vi "Control - Diesel - Cranking Host.vi"() -> ()   [LabVIEW 2015, in "ECS-Host.lvlib"]
uses:
  ECS-Host.lvlib
  <vilib>/addons/Software Calibration Management/XControls/TBL2D.xctl
panel:
  out "EngineStatus":u8
  out "_EngineStatus":enum32{"STALLED", "CRANKING", "RUNNING"}(ring)
  out "CrankModeActive":bool
  in  "ForceCrank_E":bool
  in  "Crank_E":bool
  in  "_LUT Tab":T1(tab)
  in  "InjTiming_ManE":bool
  out "InjTiming_TblOut":sgl caption="[]"
  in  "InjTiming_Man":sgl caption="[]"
  in  "InjTiming_Tbl":cluster{"X":sgl[], "Y":sgl[], "Z":sgl[][]}(xcontrol) caption="[]"
  out "InjQty_Calc":sgl caption="[]"
  in  "Phi_Max":sgl caption="[]"
  in  "InjQty_ManE":bool
  out "InjQty_TblOut":sgl caption="[]"
  in  "InjQty_Man":sgl caption="[]"
  in  "InjQty_Tbl":cluster{"X":sgl[], "Y":sgl[], "Z":sgl[][]}(xcontrol) caption="[]"
  in  "RailP_ManE":bool
  out "RailP_TblOut":sgl caption="[]"
  in  "RailP_Man":sgl caption="[]"
  in  "RailP_Tbl":cluster{"X":sgl[], "Y":sgl[], "Z":sgl[][]}(xcontrol) caption="[]"
  in  "VVTCam1Adv_ManE":bool
  out "VVTCam1Adv_TblOut":sgl caption="[]"
  in  "VVTCam1Adv_Man":sgl caption="[]"
  in  "VVTCam1Adv_Tbl":cluster{"X":sgl[], "Y":sgl[], "Z":sgl[][]}(xcontrol) caption="[]"
  in  "VVTCam2Adv_ManE":bool
  out "VVTCam2Adv_TblOut":sgl caption="[]"
  in  "VVTCam2Adv_Man":sgl caption="[]"
  in  "VVTCam2Adv_Tbl":cluster{"X":sgl[], "Y":sgl[], "Z":sgl[][]}(xcontrol) caption="[]"
  in  "VGTPsn_Crank":sgl caption="[%Open]"
  in  "WgPsn_Crank":sgl caption="[%Open]"
  in  "LowPEGRPsn_Crank":sgl caption="[%Open]"
  in  "HighPEGRPsn_Crank":sgl caption="[%Open]"
  # "(Smoke Limit)"
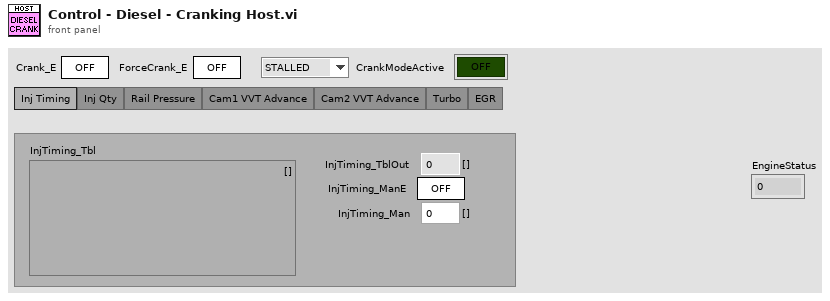
[diagram p1: front panel]
types:
  T1 = enum32{"Inj Timing", "Inj Qty", "Rail Pressure", "Cam1 VVT Advance", "Cam2 VVT Advance", "Turbo", "EGR"}
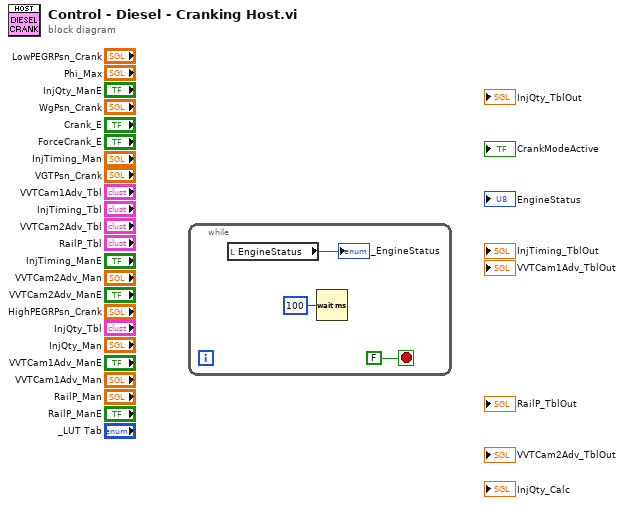
[diagram p0: block diagram]
diagram:
  n1 = while {
    stop <- FALSE stop-if-true
    n2 = local read "EngineStatus"() -> (→"_EngineStatus":u8)
    n3 = Wait (ms)(milliseconds to wait=u32 100) -> ()  [unwired: 1 out]
  }
